vi "WPI_ADI_IMU_AHRS_RoboBees.vi"(8 "Yaw Axis":enum16{"X", "Y", "Z"}(ring)=enum."Z", 10 "IMU Rates":dbl[](array[numeric])) -> (0 "Yaw":dbl(knob) scale=-180.0..180.0, 1 "Roll":dbl(knob) scale=-180.0..180.0, 2 "Pitch":dbl(knob) scale=-90.0..90.0, 3 "Output":cluster{"Pitch":dbl, "Roll":dbl, "Yaw":dbl})   [LabVIEW 2015, in "FRC ADI MXP IMU.lvlib"]
uses:
  FRC ADI MXP IMU.lvlib
panel:
  in  "Tilt Comp (Yaw)":bool=TRUE
  in  "tau mag":dbl=0.04
  in  "tau acc":dbl=0.6
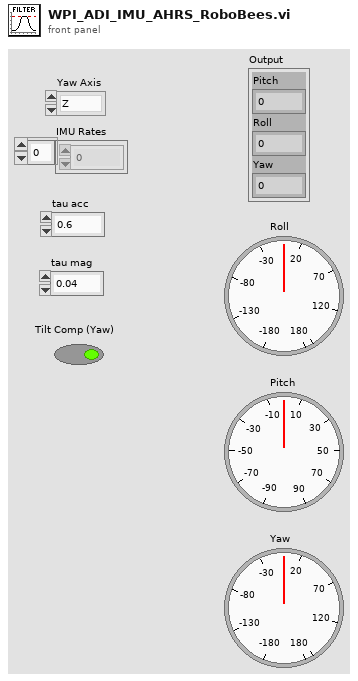
[diagram p1: front panel]
types:
  T1 = cluster{"Xaccel":dbl, "Yaccel":dbl, "Zaccel":dbl}
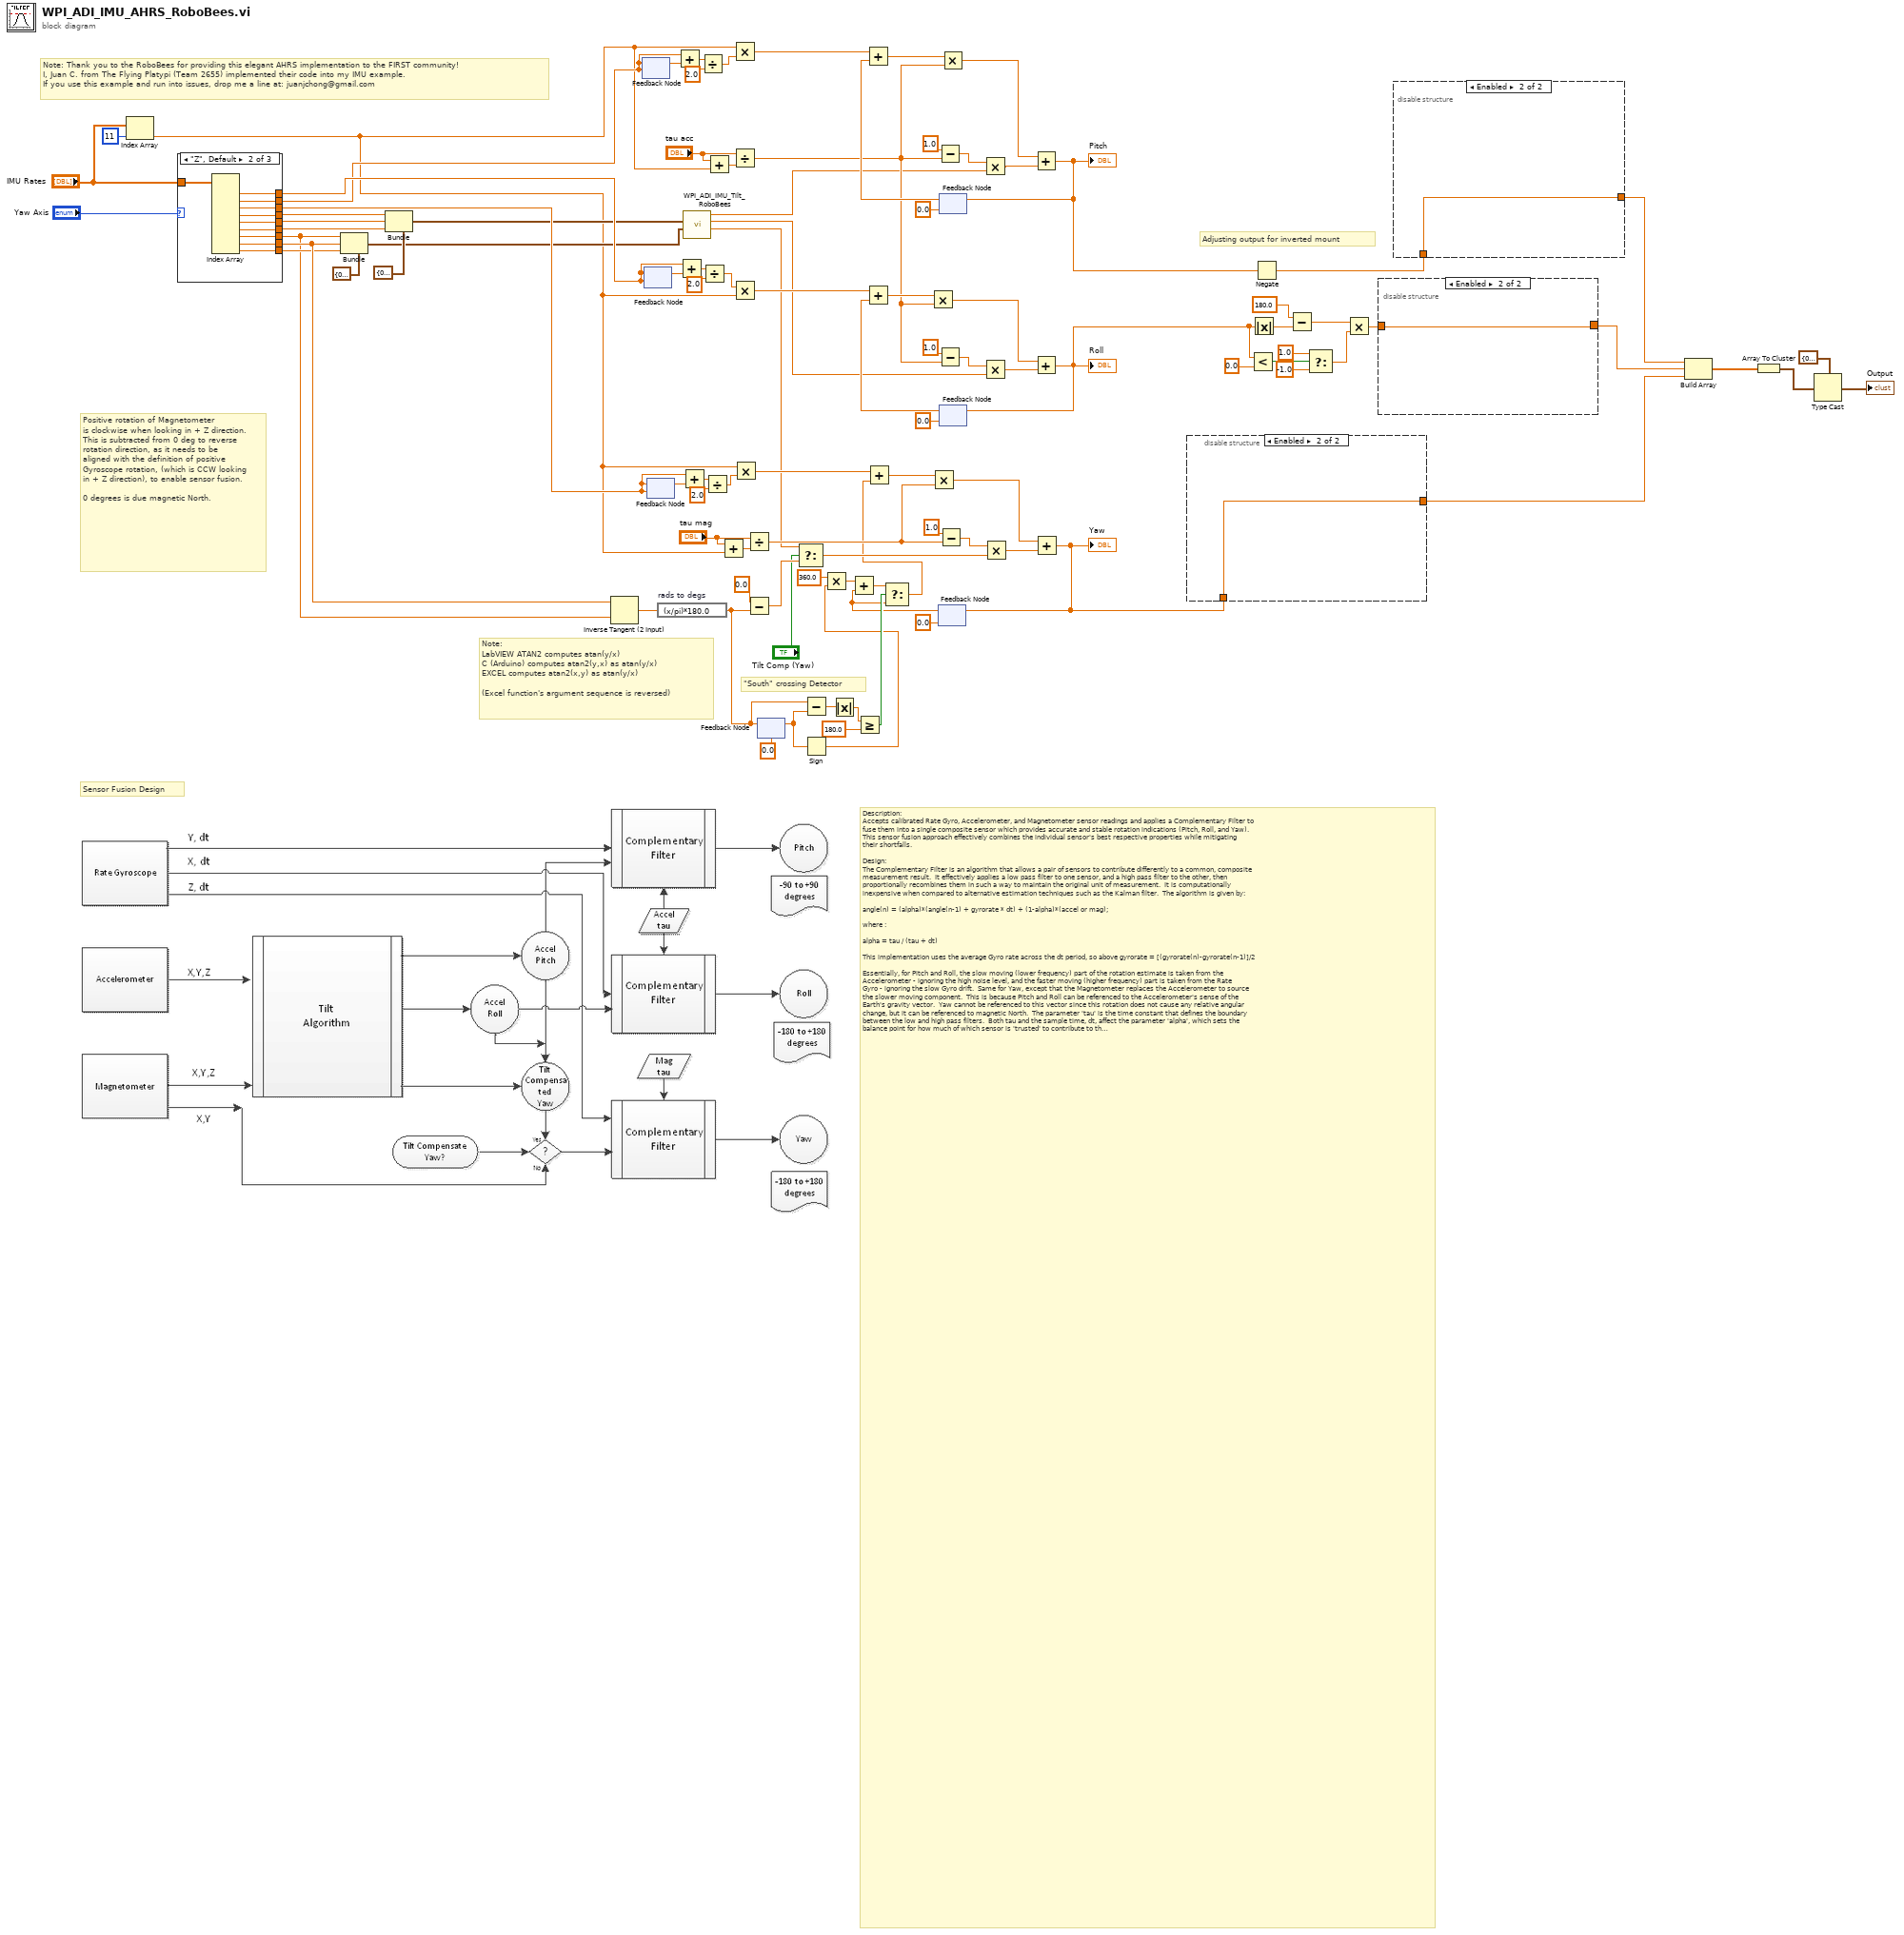
[diagram p0: block diagram]
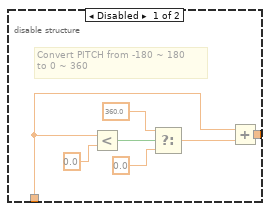
[diagram p2: hidden frame]
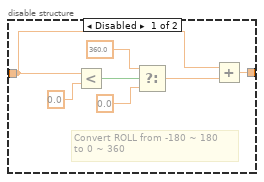
[diagram p3: hidden frame]
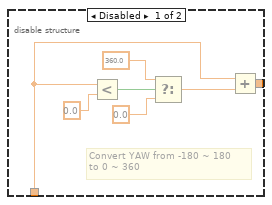
[diagram p4: hidden frame]
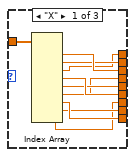
[diagram p5: hidden frame]
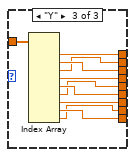
[diagram p6: hidden frame]
diagram:
  # "Note: Thank you to the RoboBees for providing this elegant AHRS implementation to the FIRST community!\nI, Juan C. from The Flying Platypi (Team 2655) implemented their code into my IMU example.\nIf you use this example and run into issues, drop me a line at: juanjchong@gmail.com"
  # "Adjusting output for inverted mount"
  # "Sensor Fusion Design"
  # "Description:\nAccepts calibrated Rate Gyro, Accelerometer, and Magnetometer sensor readings and applies a Complementary Filter to\nfuse them into a single composite sensor which provides accurate and stable rotation indications (Pitch, Roll, and Yaw).\nThis sensor fusion approach effectively combines the individual sensor's best respective properties while mitigating\ntheir shortfalls.\n\nDesign:\nThe Complementary Filter is an algorithm that allows a pair of sensors to contribute differently to a common, composite\nmeasurement result.  It effectively applies a low pass filter to one sensor, and a high pass filter to the other, then\nproportionally recombines them in such a way to maintain the original unit of measurement.  It is computationally\ninexpensive when compared to alternative estimation techniques such as the Kalman filter.  The algorithm is given by:\n\nangle(n) = (alpha)*(angle(n-1) + gyrorate * dt) + (1-alpha)*(accel or mag);\n\nwhere : \n\nalpha = tau / (tau + dt)\n\nThis implementation uses the average Gyro rate across the dt period, so above gyrorate = [(gyrorate(n)-gyrorate(n-1)]/2\n\nEssentially, for Pitch and Roll, the slow moving (lower frequency) part of the rotation estimate is taken from the\nAccelerometer - ignoring the high noise level, and the faster moving (higher frequency) part is taken from the Rate \nGyro - ignoring the slow Gyro drift.  Same for Yaw, except that the Magnetometer replaces the Accelerometer to source\nthe slower moving component.  This is because Pitch and Roll can be referenced to the Accelerometer's sense of the\nEarth's gravity vector.  Yaw cannot be referenced to this vector since this rotation does not cause any relative angular\nchange, but it can be referenced to magnetic North.  The parameter 'tau' is the time constant that defines the boundary\nbetween the low and high pass filters.  Both tau and the sample time, dt, affect the parameter 'alpha', which sets the\nbalance point for how much of which sensor is 'trusted' to contribute to the rotation estimate.\n\nThe Complementary Filter algorithm is applied to each X/Y/Z rotation axis to compute R/P/Y outputs, respectively.\n\nMagnetometer readings are tilt-compensated when Tilt-Comp-(Yaw) is asserted (True), by the IMU TILT subVI.  This\ncreates what is known as a tilt-compensated compass, which allows Yaw to be insensitive to the effects of a\nnon-level sensor, but generates error in Yaw during movement (coordinate acceleration).\n\nThe Yaw \"South\" crossing detector is necessary to allow a smooth transition across the +/- 180 deg discontinuity (inherent\nin the ATAN function).  Since -180 deg is congruent with +180 deg, Yaw needs to jump between these values when\ncrossing South (North is 0 deg).  The design depends upon comparison of successive Yaw readings to detect a cross-over\nevent.  The cross-over detector monitors the current reading and evaluates how far it is from the previous reading.  If it\nis greater than the previous reading by the Discriminant (= 180 deg), then Yaw just crossed South.\n\nBy choosing 180 as the Discriminant, the only way the detector can produce a false positive, assuming a loop iteration\nof 70 msec, is for it to rotate >2,571 dps ... (2,571=180/.07).  This is faster than the ST L3GD20 Gyro can register.  The\ndetector produces a Boolean True upon detecting a South crossing.  This is used to alter the (n-1) Yaw which was\npreviously stored, either adding or subtracting 360 degrees as required to place the previous Yaw in the correct quadrant\nwhenever crossing occurs.  The Modulus function cannot be used here as the Complementary Filter algorithm has 'state'\n(needs to remember previous Yaw).\n \nWe are in effect stitching together two ends of a ruler for 'modular arithmetic' (clock math).\n\nInputs:\nGYRO - Gyro rate and sample time measurements.\nACCEL - Acceleration measurements.\nMAG - Magnetic measurements.\nTAU ACC - tau parameter used to set sensor balance between Accel and Gyro for Roll and Pitch.\nTAU MAG -  tau parameter used to set sensor balance between Mag and Gyro for Yaw.\nTILT COMP (Yaw) - Enables Yaw tilt-compensation if True.\n\nOutputs:\nROLL - Filtered Roll about sensor X-axis.\nPITCH - Filtered Pitch about sensor Y-axis.\nYAW - Filtered Yaw about sensor Z-axis.\n\nVI Properties:\nExecution Reentrancy is set to Non Reentrant Execution\n\nImplementation:\nIt's best to establish the optimum loop sample time first.  See IMU READ implementation notes for guidance.  Each\ntau parameter should then be adjusted to achieve optimum sensor fusion.  tau acc affects Roll and Pitch, tau mag affects\nYaw.  Start at value 1 or 2 and decrease by half each time until the result doesn't drift, but not so far that the result gets\nnoisy.  An optimum tau for this IMU is likely in the range of 1.0 to 0.01, for a loop sample time between 10 and 100 ms.\n\nNote that both sample timing (dt) and tau both affect the balance parameter, 'alpha'.  Adjusting either dt or tau will\nrequire the other to be readjusted to maintain a particular filter performance.\n\nIt is likely best to set Yaw tilt-compensation to off (False) if the Yaw value is to be used as feedback in a closed loop\ncontrol application.  The tradeoff is that Yaw will only be accurate while the robot is level.\n\nSince a Yaw of -180 degrees is congruent with +180 degrees (they represent the same direction), it is possible that the\nYaw output will oscillate between these two values when the sensor happens to be pointing due South, as sensor\nnoise causes slight variation.  You will need to account for this possibility if you are using the Yaw value for decision-\nmaking in code.\n\n----- The RoboBees FRC Team 836! -----  Complement your passion to solve problems with a STEM Education!"
  # "\"South\" crossing Detector"
  # "Positive rotation of Magnetometer\nis clockwise when looking in + Z direction.  This is subtracted from 0 deg to reverse rotation direction, as it needs to be aligned with the definition of positive Gyroscope rotation, (which is CCW looking in + Z direction), to enable sensor fusion.\n\n0 degrees is due magnetic North."
  # "Note:\nLabVIEW ATAN2 computes atan(y/x)\nC (Arduino) computes atan2(y,x) as atan(y/x)\nEXCEL computes atan2(x,y) as atan(y/x)\n\n(Excel function's argument sequence is reversed)"
  n1 = Index Array(array="IMU Rates", index=11) -> (element=w5:dbl)
  n2 = case shown="\"Z\", Default" "Yaw Axis" {
    tunnel: [w106 w119 w128] -> w39
    tunnel: [w103 w118 w125] -> w32
    tunnel: "IMU Rates" -> [w109 w117 w129]
    tunnel: [w100 w116 w122] -> w34
    tunnel: [w104 w115 w123] -> w31
    tunnel: [w105 w114 w124] -> w30
    tunnel: [w107 w113 w126] -> w38
    tunnel: [w108 w112 w127] -> w37
    tunnel: [w101 w111 w120] -> w36
    tunnel: [w102 w110 w121] -> w35
    frame "X" {
      n3 = Index Array(array=w109) -> (element #1=w108:dbl, element #2=w107:dbl, element #3=w106:dbl, element #4=w105:dbl, element #5=w104:dbl, element #6=w103:dbl, element #7=w102:dbl, element #8=w101:dbl, element #9=w100:dbl)  [unwired: 9 in]
    }
    frame "Z", Default {
      n4 = Index Array(array=w117) -> (element #1=w119:dbl, element #2=w113:dbl, element #3=w112:dbl, element #4=w118:dbl, element #5=w115:dbl, element #6=w114:dbl, element #7=w116:dbl, element #8=w111:dbl, element #9=w110:dbl)  [unwired: 9 in]
    }
    frame "Y" {
      n5 = Index Array(array=w129) -> (element #1=w128:dbl, element #2=w127:dbl, element #3=w126:dbl, element #4=w125:dbl, element #5=w124:dbl, element #6=w123:dbl, element #7=w122:dbl, element #8=w121:dbl, element #9=w120:dbl)  [unwired: 9 in]
    }
  }
  n6 = Bundle(cluster=cluster{"Xmag":dbl, "Ymag":dbl, "Zmag":dbl} {"Xmag"=0.0, "Ymag"=0.0, "Zmag"=0.0} ("Mag"), "Xmag"=w34, "Ymag"=w36, "Zmag"=w35) -> (w27:cluster{"Xmag":dbl, "Ymag":dbl, "Zmag":dbl})
  n7 = Bundle(cluster=T1 {"Xaccel"=0.0, "Yaccel"=0.0, "Zaccel"=0.0} ("Accel"), "Xaccel"=w32, "Yaccel"=w31, "Zaccel"=w30) -> (w28:T1)
  n8 = Inverse Tangent (2 Input)(1:w34, 2:w36) -> (0:w72:dbl)
  n9 = feedback #1(w38) -> (w61:dbl)
  n10 = feedback-in #1(w38) -> ()
  n11 = feedback #2(w39) -> (w55:dbl)
  n12 = feedback-in #2(w39) -> ()
  n13 = feedback #3(w37) -> (w53:dbl)
  n14 = feedback-in #3(w37) -> ()
  n15 = expression code="(x/pi)*180.0" "rads to degs"(w72) -> (w42:dbl)
  n16 = Add(x=w38, y=w61) -> (x+y=w60:dbl)
  n17 = Add(x=w39, y=w55) -> (x+y=w56:dbl)
  n18 = Add(x=w37, y=w53) -> (x+y=w52:dbl)
  n19 = call "WPI_ADI_IMU_Tilt_RoboBees.vi"("Mag"=w27, "Accel"=w28) -> ("Yaw"=w24:dbl, "Roll"=w25:dbl, "Pitch"=w26:dbl)  [unwired: 6 in, 1 out]
  n20 = Divide(x=w60, y=2.0) -> (x/y=w58:dbl)
  n21 = Divide(x=w56, y=2.0) -> (x/y=w54:dbl)
  n22 = Divide(x=w52, y=2.0) -> (x/y=w50:dbl)
  n23 = Add(x="tau acc", y=w5) -> (x+y=w98:dbl)
  n24 = Add(x="tau mag", y=w5) -> (x+y=w73:dbl)
  n25 = Multiply(x=w5, y=w58) -> (x*y=w86:dbl)
  n26 = Divide(x="tau acc", y=w98) -> (x/y=w82:dbl)
  n27 = Multiply(x=w54, y=w5) -> (x*y=w96:dbl)
  n28 = Multiply(x=w5, y=w50) -> (x*y=w66:dbl)
  n29 = Divide(x="tau mag", y=w73) -> (x/y=w65:dbl)
  n30 = Subtract(x=0.0 ("y"), y=w42) -> (x-y=w69:dbl)
  n31 = feedback #4(0.0) -> (w43:dbl)
  n32 = feedback-in #4(w42) -> ()
  n33 = Select(t=w24, s="Tilt Comp (Yaw)", f=w69) -> (s? t:f=w70:dbl)
  n34 = Subtract(x=w42, y=w43) -> (x-y=w49:dbl)
  n35 = Sign(1:w43) -> (0:w45:dbl)
  n36 = Multiply(x=360.0 ("y"), y=w45) -> (x*y=w41:dbl)
  n37 = Absolute Value(x=w49) -> (abs(x)=w48:dbl)
  n38 = Greater Or Equal?(x=w48, y=180.0) -> (x >= y?=w46:bool)
  n39 = Subtract(x=1.0, y=w82) -> (x-y=w85:dbl)
  n40 = Subtract(x=1.0, y=w82) -> (x-y=w81:dbl)
  n41 = Subtract(x=1.0, y=w65) -> (x-y=w79:dbl)
  n42 = feedback #5(0.0) -> (w40:dbl)
  n43 = Add(x=w41, y=w40) -> (x+y=w62:dbl)
  n44 = Select(t=w62, s=w46, f=w40) -> (s? t:f=w63:dbl)
  n45 = Add(x=w66, y=w63) -> (x+y=w76:dbl)
  n46 = Multiply(x=w76, y=w65) -> (x*y=w78:dbl)
  n47 = feedback #6(0.0) -> (w90:dbl)
  n48 = Add(x=w86, y=w90) -> (x+y=w87:dbl)
  n49 = Multiply(x=w87, y=w82) -> (x*y=w89:dbl)
  n50 = feedback #7(0.0) -> (w80:dbl)
  n51 = Add(x=w96, y=w80) -> (x+y=w95:dbl)
  n52 = Multiply(x=w95, y=w82) -> (x*y=w93:dbl)
  n53 = Multiply(x=w85, y=w26) -> (x*y=w88:dbl)
  n54 = Multiply(x=w81, y=w25) -> (x*y=w94:dbl)
  n55 = Multiply(x=w79, y=w70) -> (x*y=w77:dbl)
  n56 = Add(x=w89, y=w88) -> (x+y=w15:dbl)
  "Pitch" <- w15
  n57 = feedback-in #6(w15) -> ()
  n58 = Add(x=w93, y=w94) -> (x+y=w14:dbl)
  "Roll" <- w14
  n59 = feedback-in #7(w14) -> ()
  n60 = Add(x=w78, y=w77) -> (x+y=w13:dbl)
  "Yaw" <- w13
  n61 = feedback-in #5(w13) -> ()
  n62 = disable-structure shown="Enabled" {
    disable-tunnel: w13 -> [w131 w137]
    disable-tunnel: [w130 w137] -> w12
    frame Disabled {
      # "Convert YAW from -180 ~ 180 \nto 0 ~ 360"
      n63 = Less?(x=w131, y=0.0) -> (x < y?=w135:bool)
      n64 = Select(t=360.0, s=w135, f=0.0) -> (s? t:f=w132:dbl)
      n65 = Add(x=w131, y=w132) -> (x+y=w130:dbl)
    }
    frame Enabled {
    }
  }
  n66 = Less?(x=w14, y=0.0) -> (x < y?=w20:bool)
  n67 = Absolute Value(x=w14) -> (abs(x)=w23:dbl)
  n68 = Negate(x=w15) -> (-x=w8:dbl)
  n69 = Subtract(x=180.0 ("y"), y=w23) -> (x-y=w17:dbl)
  n70 = Select(t=1.0, s=w20, f=-1.0) -> (s? t:f=w16:dbl)
  n71 = Multiply(x=w17, y=w16) -> (x*y=w11:dbl)
  n72 = disable-structure shown="Enabled" {
    disable-tunnel: w11 -> [w139 w145]
    disable-tunnel: [w138 w145] -> w10
    frame Disabled {
      # "Convert ROLL from -180 ~ 180 \nto 0 ~ 360"
      n73 = Less?(x=w139, y=0.0) -> (x < y?=w143:bool)
      n74 = Select(t=360.0, s=w143, f=0.0) -> (s? t:f=w140:dbl)
      n75 = Add(x=w139, y=w140) -> (x+y=w138:dbl)
    }
    frame Enabled {
    }
  }
  n76 = disable-structure shown="Enabled" {
    disable-tunnel: [w147 w153] -> w9
    disable-tunnel: w8 -> [w146 w153]
    frame Disabled {
      # "Convert PITCH from -180 ~ 180 \nto 0 ~ 360"
      n77 = Less?(x=w146, y=0.0) -> (x < y?=w151:bool)
      n78 = Select(t=360.0, s=w151, f=0.0) -> (s? t:f=w148:dbl)
      n79 = Add(x=w146, y=w148) -> (x+y=w147:dbl)
    }
    frame Enabled {
    }
  }
  n80 = Build Array(w9, w10, w12) -> (w2:dbl[])
  n81 = Array To Cluster(array=w2) -> (cluster=w3:cluster{"[0]":dbl, "[1]":dbl, "[2]":dbl})
  n82 = Type Cast(type=cluster{"Pitch":dbl, "Roll":dbl, "Yaw":dbl} {"Pitch"=0.0, "Roll"=0.0, "Yaw"=0.0} ("IMU AHRS"), x=w3) -> (*(type *) &x=→"Output":cluster{"Pitch":dbl, "Roll":dbl, "Yaw":dbl})
